vi "Create Q.vi"(8 "error in (no error)":errorcluster) -> (0 "error out":errorcluster)   [LabVIEW 2017, in "Messaging Library.lvlib"]
uses:
  Messaging Library.lvlib
  Controls/Msg TypeDef.ctl
  Controls/Q FGV States.ctl
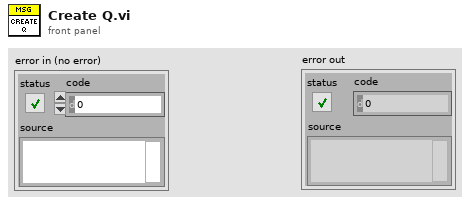
[diagram p1: front panel]
types:
  T1 = typedef "Messaging Library.lvlib/Q FGV States.ctl" = enum16{"Set", "Get"}
  T2 = typedef "Messaging Library.lvlib/Msg TypeDef.ctl" = cluster{"Message":string, "Data":variant}
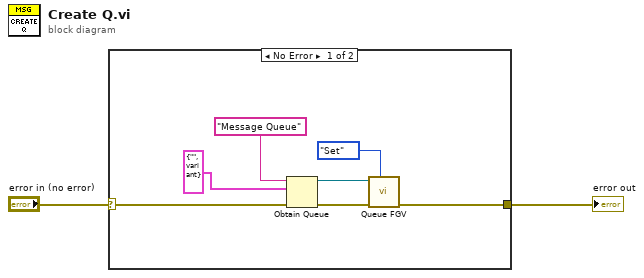
[diagram p0: block diagram]
diagram:
  n1 = case shown="No Error" "error in (no error)" {
    selector: "error in (no error)" -> [w9 w10]
    tunnel: [w4 w10] -> w1
    frame No Error {
      n2 = Obtain Queue(name (unnamed)="Message Queue", element data type=T2 {"Message"="", "Data"=variant} ("Message Cluster"), error in (no error)=w9) -> (queue out=w6:refnum<queue>, error out=w5:errorcluster)  [unwired: 2 in, 1 out]
      n3 = call "Queue FGV.vi"("States"=Q_FGV_States."Set", "error in (no error)"=w5, "Message Q In"=w6) -> ("error out"=w4:errorcluster)  [unwired: 7 in, 1 out]
    }
    frame Error {
    }
  }
  "error out" <- w1
